vi "Get Desired Size.vi"(8 "error in (no error)":errorcluster, 11 "Element A in":refnum<class "Element B.lvclass">) -> (0 "error out":errorcluster, 2 "Desired Size":T1, 3 "Element A out":refnum<class "Element B.lvclass">)   [LabVIEW 2020, in "Array Example.lvlib" / "Element B.lvclass"]
uses:
  Element B.lvclass
  OOPanel/ArrayPanel/Desired Size.ctl
  OOPanel/OOPanel.lvlib
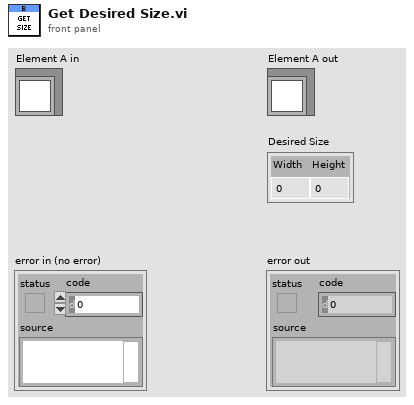
[diagram p1: front panel]
types:
  T1 = typedef "OOPanel.lvlib/Desired Size.ctl" = cluster{"Width":u32, "Height":u32}
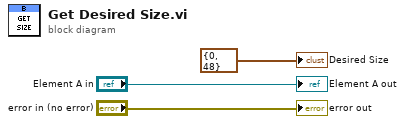
[diagram p0: block diagram]
diagram:
  "error out" <- "error in (no error)"
  "Element A out" <- "Element A in"
  "Desired Size" <- T1 {"Width"=0, "Height"=48} ("Desired Size")
